vi "Prep to Fire.vi"(9 "Fully down?":bool, 11 "Input":bool) -> (3 "Latched":bool)   [LabVIEW 2013]
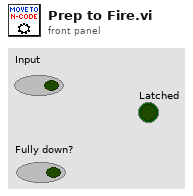
[diagram p1: front panel]
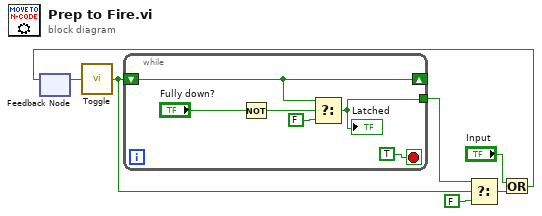
[diagram p0: block diagram]
diagram:
  n1 = feedback #1() -> (w4:bool)  [unwired: 1 in]
  n2 = call "Toggle.vi"("Input"=w4) -> ("Latched"=w1:bool)
  n3 = while {
    shift-right: [w12] -> _
    shift-left: w1 -> [w12]
    tunnel: [w11] -> w2
    stop <- TRUE stop-if-true
    n4 = Not(x="Fully down?") -> (.not. x?=w9:bool)
    n5 = Select(t=w12, s=w9, f=FALSE) -> (s? t:f=w11:bool)
    "Latched" <- w11
  }
  n6 = Select(t=w2, s=w1, f=FALSE) -> (s? t:f=w6:bool)
  n7 = Or(x="Input", y=w6) -> (x .or. y?=w5:bool)
  n8 = feedback-in #1(w5) -> ()
